vi "SetImageType.vi"(8 "error in (no error)":errorcluster, 10 "ImageType":T1, 11 "CameraTestingProxyAPI in":refnum<class "CameraTestingProxyAPI.lvclass">) -> (0 "error out":errorcluster, 3 "CameraTestingProxyAPI out":refnum<class "CameraTestingProxyAPI.lvclass">)   [LabVIEW 2020, in "CameraTestingProxy.lvlib" / "CameraTestingProxyAPI.lvclass"]
uses:
  CameraTestingProxyAPI.lvclass
  ICameraTestingProxy/ICameraTestingProxy/TypeDef/ImageType.ctl
  ICameraTestingProxy/ICameraTestingProxy/TypeDef/Color Model.ctl
  CameraTestingProxyAPI.lvclass/CameraTestingProxyAPI.ctl
  95c060c7-3025-4c1d-be19-476899711a5a.vi
  ICameraTestingProxy/ICameraTestingProxy/ICameraTestingProxy.lvclass
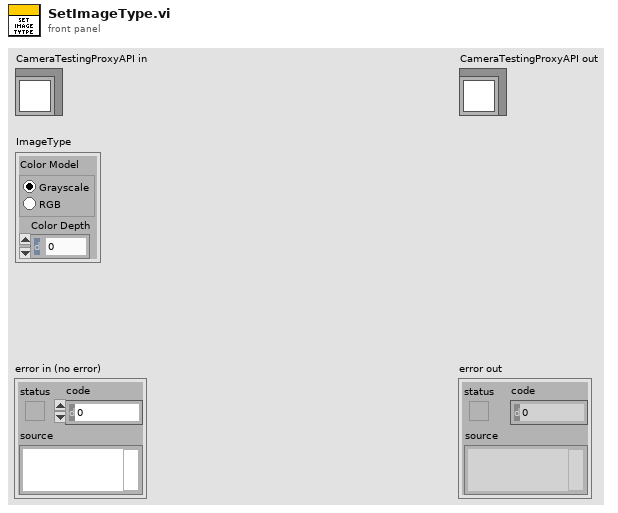
[diagram p1: front panel]
types:
  T1 = typedef "ICameraTestingProxy.lvlib/ICameraTestingProxy.lvclass/ImageType.ctl" = cluster{"Color Model":T2, "Color Depth":u8}
  T2 = typedef "ICameraTestingProxy.lvlib/ICameraTestingProxy.lvclass/Color Model.ctl" = enum32{"Grayscale", "RGB"}
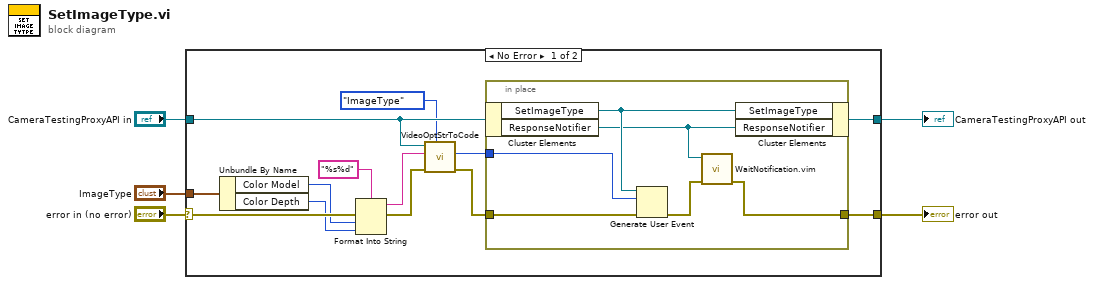
[diagram p0: block diagram]
diagram:
  n1 = case shown="No Error" "error in (no error)" {
    selector: "error in (no error)" -> [w13 w26]
    tunnel: "CameraTestingProxyAPI in" -> [w16 w25]
    tunnel: [w18 w26] -> w2
    tunnel: [w17 w25] -> w4
    tunnel: "ImageType" -> [w10 _]
    frame No Error {
      n2 = Unbundle By Name(w10) -> ("Color Model"=w9:T2, "Color Depth"=w8:u8)
      n3 = Format Into String(format string="%s%d", error in=w13, w9, w8) -> (resulting string=w14:string, error out=w12:errorcluster)  [unwired: 1 in]
      n4 = call "VideoOptStrToCode.vi"("VideoOption"=enum16{"FrameRate", "ImageType", "Resolution"}."ImageType", "error in (no error)"=w12, "DescriptionString"=w14, "CameraTestingProxyAPI in"=w16) -> ("error out"=w11:errorcluster, "Code"=w15:u8)  [unwired: 5 in, 1 out]
      n5 = in-place {
        in-place-border: w11 -> [w24]
        in-place-border: [w19] -> w18
        in-place-border: w15 -> [w22]
        n6 = in-place-cluster #1(w16) -> ("SetImageType"=w23:refnum<user-event>, "ResponseNotifier"=w21:refnum<notifier>)
        n7 = Generate User Event(user event=w23, event data cluster=w22, error in=w24) -> (error out=w20:errorcluster)  [unwired: 1 in, 1 out]
        n8 = call "WaitNotification.vim"("error in (no error)"=w20, "ResponseNotifier"=w21) -> ("error out"=w19:errorcluster)  [unwired: 8 in, 1 out]
        n9 = in-place-cluster #1("SetImageType"=w23, "ResponseNotifier"=w21) -> (w17:refnum<class "CameraTestingProxyAPI.lvclass">)
      }
    }
    frame Error {
    }
  }
  "error out" <- w2
  "CameraTestingProxyAPI out" <- w4
